vi "Set Measurement Properties.vi"(6 "Measurement Type":T1=10 items=["Continuity", "Current AC", "Current DC", "Diode", "Frequency", "Resistance 4-wire", "Period", "Resistance 2-wire", "Temperature", "Voltage AC", "Voltage DC", "Voltage DC Ratio", "Capacitance"], 7 "Auto Range":bool, 8 "error in (no error)":errorcluster, 9 "Manual Resolution":dbl=1e-05 format="%#_6e", 10 "Manual Range":dbl=1.0, 11 "34401 in":refnum<class "34401.lvclass">) -> (0 "error out":errorcluster, 3 "34401 out":refnum<class "34401.lvclass">)   [LabVIEW 2018, in "34401.lvlib" / "34401.lvclass"]
uses:
  34401.lvclass
  PPLs/DMM/Parent/DMM.lvlibp/Custom Controls/Measurement Type.ctl
  34401.lvclass/34401.ctl
  PPLs/DMM/Parent/DMM.lvlibp/DMM.lvclass
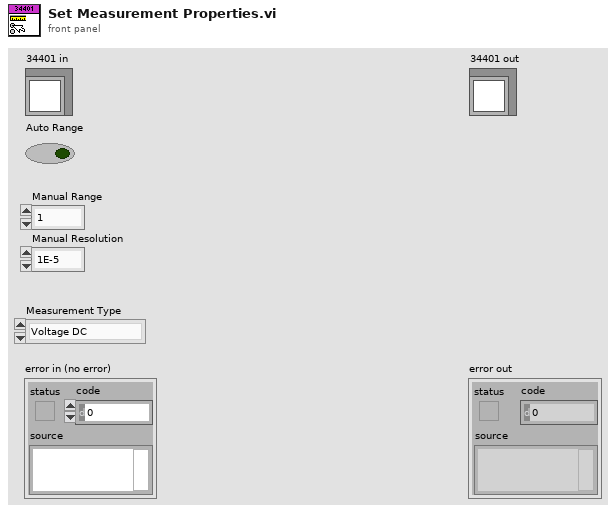
[diagram p1: front panel]
types:
  T1 = typedef "DMM.lvlibp/DMM.lvclass/Measurement Type.ctl" = u32
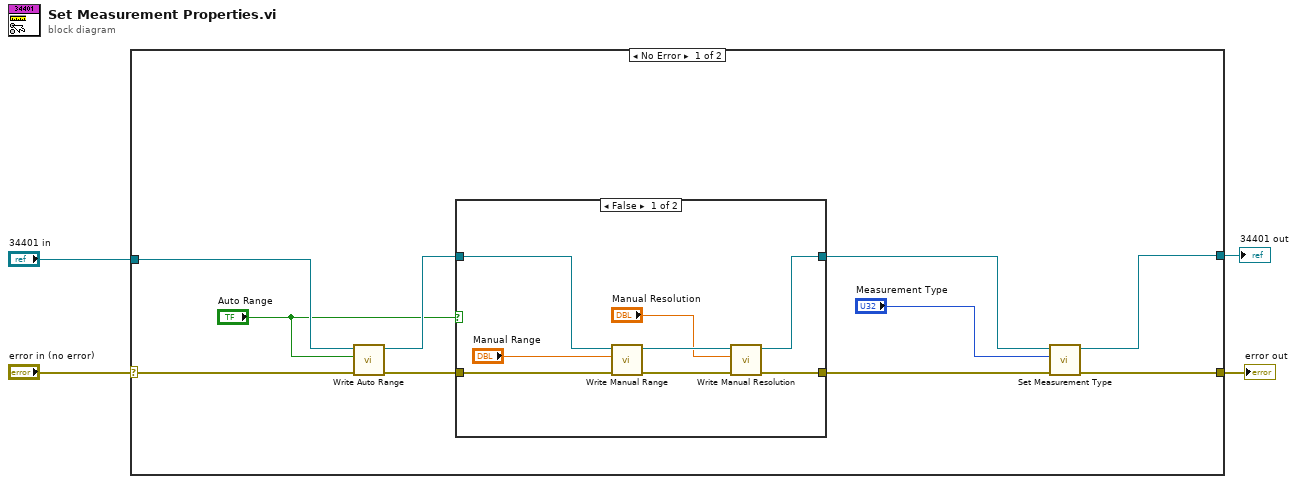
[diagram p0: block diagram]
diagram:
  n1 = case shown="No Error" "error in (no error)" {
    selector: "error in (no error)" -> [w13 w26]
    tunnel: [w6 w26] -> w3
    tunnel: [w5 w25] -> w1
    tunnel: "34401 in" -> [w12 w25]
    frame No Error {
      n2 = call "Write Auto Range.vi"("error in (no error)"=w13, "Auto Range"="Auto Range", "34401 in"=w12) -> ("error out"=w8:errorcluster, "34401 out"=w11:refnum<class "34401.lvclass">)  [unwired: 7 in]
      n3 = case shown="False" "Auto Range" {
        tunnel: w11 -> [w20 w24]
        tunnel: [w18 w24] -> w9
        tunnel: w8 -> [w22 w23]
        tunnel: [w15 w23] -> w7
        frame False {
          n4 = call "Write Manual Range.vi"("error in (no error)"=w22, "Manual Range"="Manual Range", "34401 in"=w20) -> ("error out"=w21:errorcluster, "34401 out"=w19:refnum<class "34401.lvclass">)  [unwired: 7 in]
          n5 = call "Write Manual Resolution.vi"("error in (no error)"=w21, "Manual Resolution"="Manual Resolution", "34401 in"=w19) -> ("error out"=w15:errorcluster, "34401 out"=w18:refnum<class "34401.lvclass">)  [unwired: 7 in]
        }
        frame True {
        }
      }
      n6 = call-dynamic "Set Measurement Type.vi"("error in (no error)"=w7, "Measurement Type"="Measurement Type", "34401 in"=w9) -> ("error out"=w6:errorcluster, "34401 out"=w5:refnum<class "34401.lvclass">)  [unwired: 7 in]
    }
    frame Error {
    }
  }
  "error out" <- w3
  "34401 out" <- w1
